vi "Manual Override Requested (Deprecated).vi"(10 "Is Idle?":bool, 11 "Operator Buttons":bool[](array[boolean])) -> (3 "Manual Override Requested?":bool)   [LabVIEW 2020]
uses:
  <vilib>/Rock Robotics/WPI/Joystick/XBox Buttons Indexer.ctl
  4066c891-66c7-47f2-8b8c-f67443423b77.vi
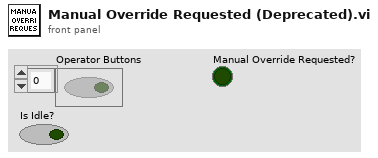
[diagram p1: front panel]
types:
  T1 = typedef "XBox Buttons Indexer.ctl" = enum16{"A", "B", "X", "Y", "Left Bumper", "Right Bumper", "Back", "Start", "Left Joystick", "Right Joystick"}
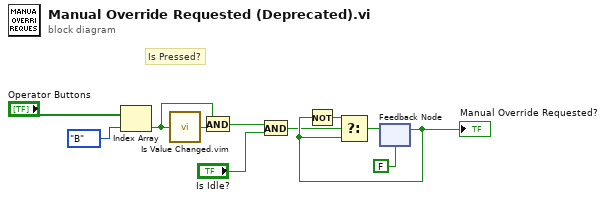
[diagram p0: block diagram]
diagram:
  # "Is Pressed?"
  n1 = Index Array(array="Operator Buttons", index=XBox_Buttons_Indexer."B" ("XBox Buttons")) -> (element=w8:bool)
  n2 = call "Is Value Changed.vim"("value"=w8) -> ("changed or first call?"=w9:bool)
  n3 = And(x=w8, y=w9) -> (x .and. y?=w3:bool)
  n4 = And(x=w3, y="Is Idle?") -> (x .and. y?=w1:bool)
  n5 = feedback #1(FALSE) -> (w4:bool)
  "Manual Override Requested?" <- w4
  n6 = Not(x=w4) -> (.not. x?=w5:bool)
  n7 = Select(t=w5, s=w1, f=w4) -> (s? t:f=w6:bool)
  n8 = feedback-in #1(w6) -> ()
